vi "Actor Core.vi"(8 "error in":errorcluster, 11 "CS++MCSGui.lvclass":refnum<class "CS++MCSGui.lvclass">) -> (0 "Error Out":errorcluster, 3 "Actor out":refnum<class "Actor.lvclass">)   [LabVIEW 2016, in "CS++MCSGui.lvlib" / "CS++MCSGui.lvclass"]
doc: "(<B>Filename</B>: Actor Framework.lvlib:Actor.lvclass:Actor Core.vi)\n\nReceives messages to the actor, reacts to them, and initiates any error handling that may shut the actor down.\n\nDescendant classes may override this VI to append parallel tasks for the actor to complete while it handles messages. Overrides use the Call Parent Method node."
uses:
  CS++MCSGui.lvclass
  C:/User/Brand/LVP/CSPP-Dev/Packages/CSPP_Core/Actors/CS++BaseActor/CS++BaseActor.lvclass
  C:/User/Brand/LVP/CSPP-Dev/Packages/CSPP_Core/Actors/CS++GUIActor/CS++GUIActor.lvclass
  C:/Program Files (x86)/National Instruments/LabVIEW 2016/vi.lib/ActorFramework/Actor/Actor.lvclass
  <vilib>/ActorFramework/Actor/Actor.lvclass
  CSPP_Core/Actors/CS++BaseActor/CS++BaseActor.lvclass/CS++BaseActor.ctl
  CSPP_Core/Actors/CS++GUIActor/CS++GUIActor.lvclass/CS++GUIActor.ctl
  <vilib>/ActorFramework/Actor/Actor.lvclass/Actor.ctl
  <vilib>/ActorFramework/Message Enqueuer/Message Enqueuer.lvclass/Message Enqueuer.ctl
  CSPP_Core/Classes/CS++ProcessVariables/ProcessVariable/PV.lvclass/PV.ctl
  CSPP_Core/Actors/CS++BaseActor/Read Object Name.vi
  CSPP_Core/Actors/CS++BaseActor/Read CS++Factory.vi
  CSPP_Core/Actors/CS++GUIActor/Read Associated Actor Name.vi
  CSPP_Core/Classes/CS++ProcessVariables/ProcessVariable/Read Data.vi
  CSPP_Core/Classes/CS++ProcessVariables/ProcessVariable/Read Name.vi
  CSPP_Core/Classes/CS++ProcessVariables/ProcessVariable/Read Timestamp.vi
  CSPP_Core/Actors/CS++GUIActor/Read Stop-Event.vi
  CSPP_Core/Actors/CS++GUIActor/Read PV-Update.vi
  CSPP_Core/Actors/CS++GUIActor/Read Associated Proxy Actor Enqueuer.vi
  <vilib>/ActorFramework/Message Enqueuer/Init from Existing Queue.vi
  <vilib>/ActorFramework/Message Enqueuer/Enqueue.vi
  <vilib>/ActorFramework/Stop Msg/Stop Msg.lvclass
  C:/Program Files (x86)/National Instruments/LabVIEW 2016/vi.lib/ActorFramework/Message/Message.lvclass
  <vilib>/ActorFramework/Message Priority Queue/Priority Enqueue.vi
  CSPP_Core/Classes/CS++ProcessVariables/PVConnection/PVConnection.lvclass
  CSPP_Core/Classes/CS++BaseClasses/Factory/CS++Factory.lvclass
  CSPP_Core/Classes/CS++ProcessVariables/ProcessVariable/PV.lvclass
  <vilib>/ActorFramework/Message Enqueuer/Message Enqueuer.lvclass
  CSPP_Core/Actors/CS++DeviceGUIActor/CS++DeviceGUIActor.lvclass
  CSPP_Core/Actors/CS++BaseActor/CS++BaseActor.lvclass
  CSPP_Core/Actors/CS++GUIActor/CS++GUIActor.lvclass
  CSPP_Core/Libraries/Utilities/CS++Utilities.lvlib
panel:
  in  "Tab Control":enum32{"Info", "Configuration", "Measurement"}(tab)
  out "Last Update":timestamp
  out "Associated Device Actor":string
  out "Resource Name":string
  out "Self-Test Result Message":string
  out "Self-Test Result Code":i32
  out "Firmware Revision":string
  out "Driver Revision":string
  in  "Read Button":bool
  in  "TriggerSlope":u16(ring) items=["rising", "falling"]
  in  "DiscriminatorSlope":u16(ring) items=["rising", "falling"]
  out "Actual Bin Width":dbl[unit]
  in  "NumberOfRecords":dbl
  in  "NumberOfBins":dbl
  in  "Bin Width":dbl[unit]
  in  "Trigger Level":dbl[unit]
  in  "Discriminator Level":dbl[unit]
  in  "Read Button":bool
  out "Status":dbl
  in  "Clear Button":bool
  in  "Stop Button":bool
  in  "Start Button":bool
  out "TotalCounts":dbl
  out "Counts":dbl
  out "NumberOfBins":dbl
  out "NumberOfRecords":dbl
  out "Bin Width":dbl[unit]
  out "Waveform Graph":dbl[](graph)
  in  "Stop Button":bool
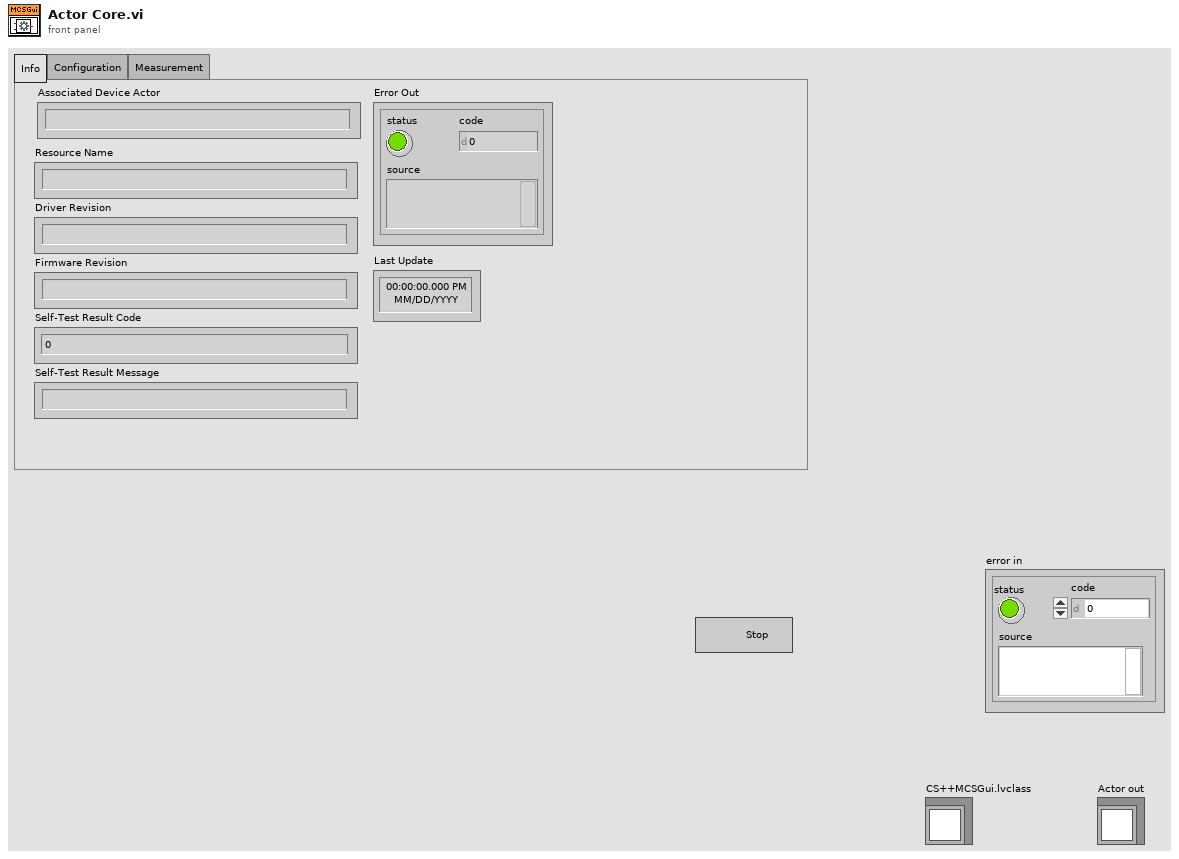
[diagram p1: front panel]
types:
  T1 = enum32{"Invalid", "Standard", "Closed", "Hidden", "Minimized", "Maximized"}
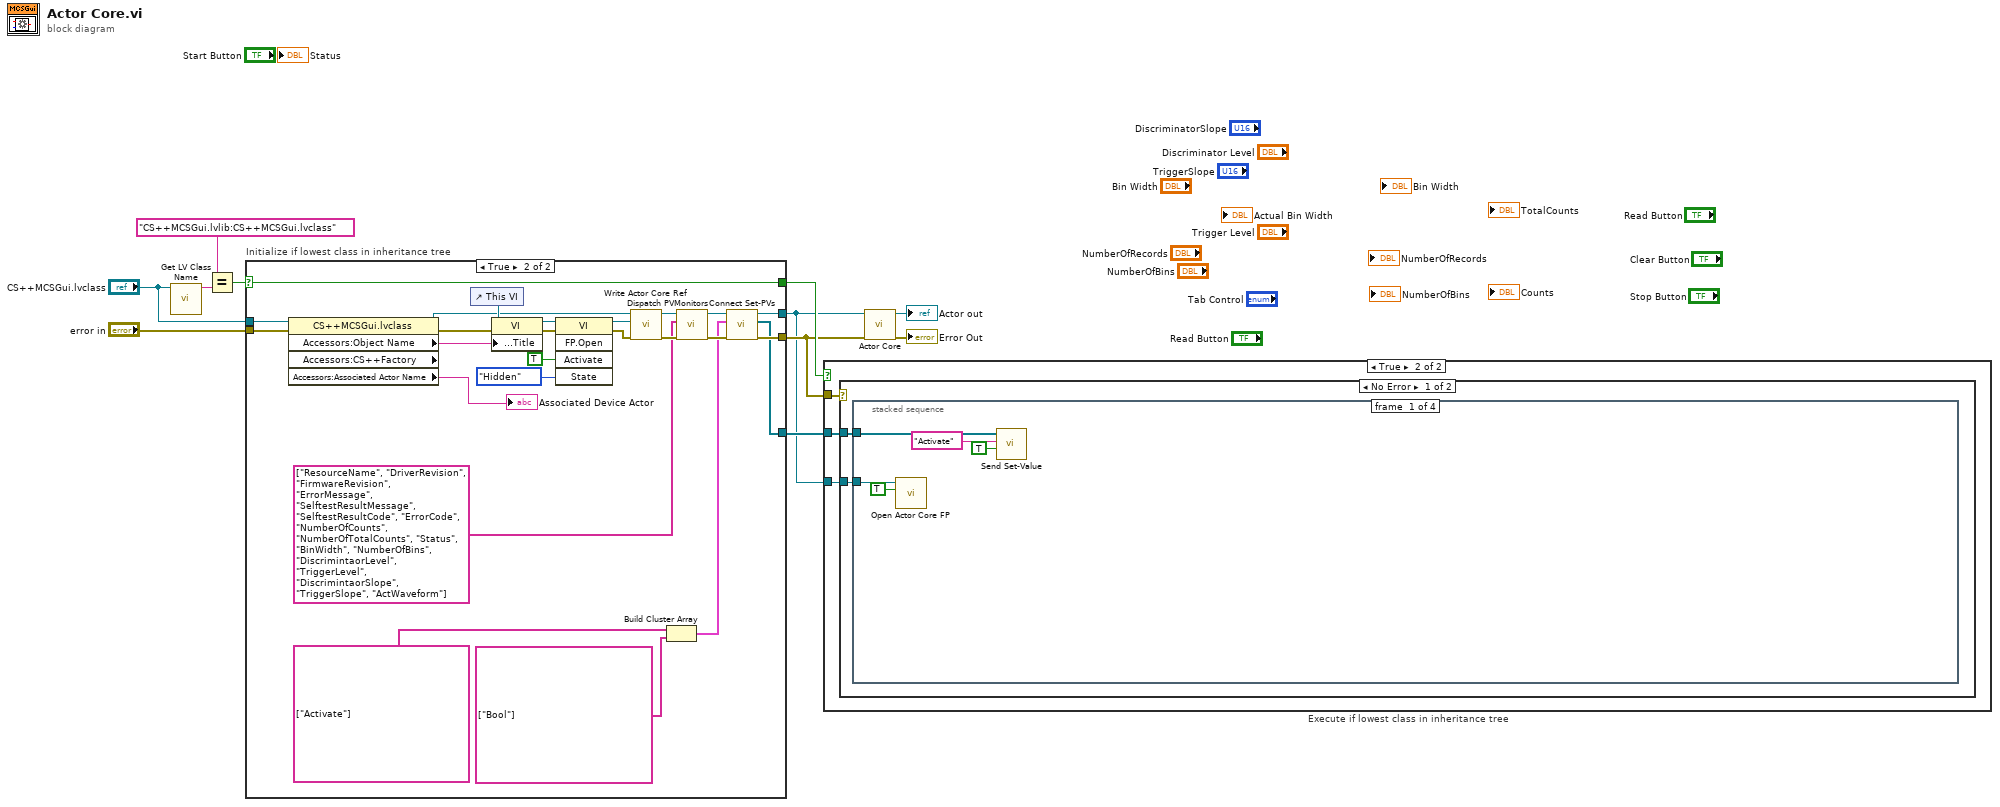
[diagram p0: block diagram]
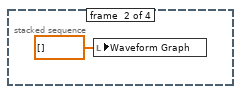
[diagram p3: hidden frame]
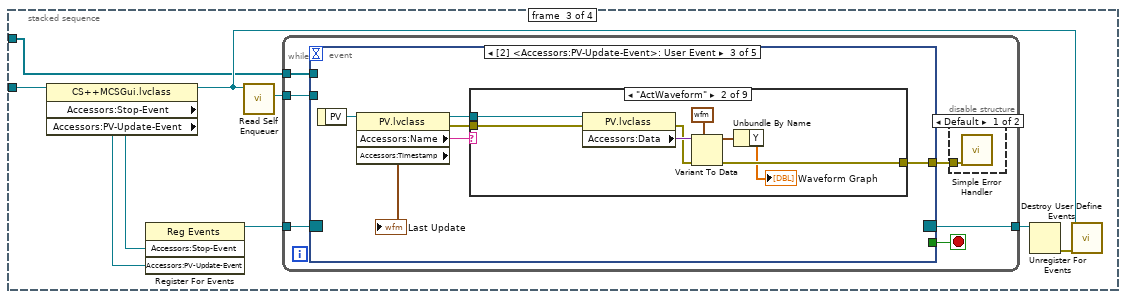
[diagram p4: hidden frame]
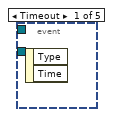
[diagram p6: hidden frame]
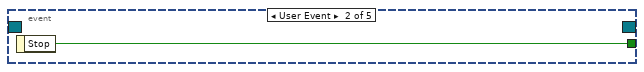
[diagram p7: hidden frame]
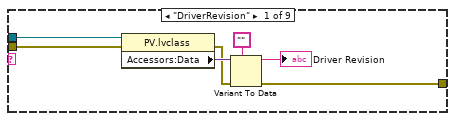
[diagram p8: hidden frame]
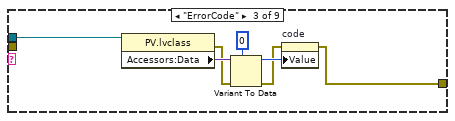
[diagram p9: hidden frame]
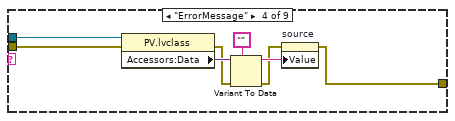
[diagram p10: hidden frame]
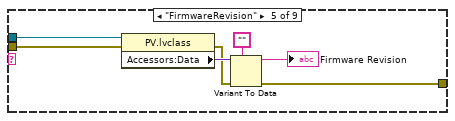
[diagram p11: hidden frame]
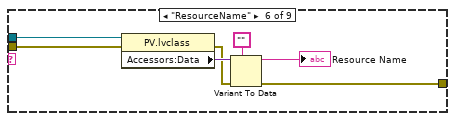
[diagram p12: hidden frame]
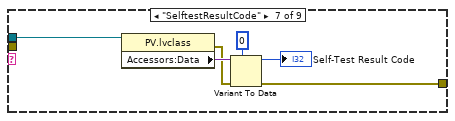
[diagram p13: hidden frame]
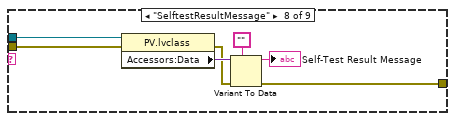
[diagram p14: hidden frame]
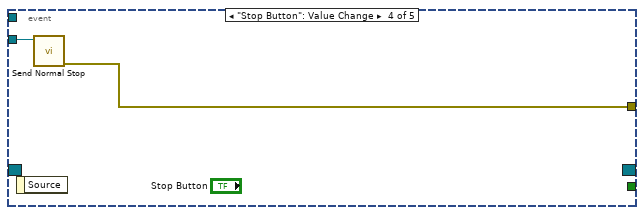
[diagram p16: hidden frame]
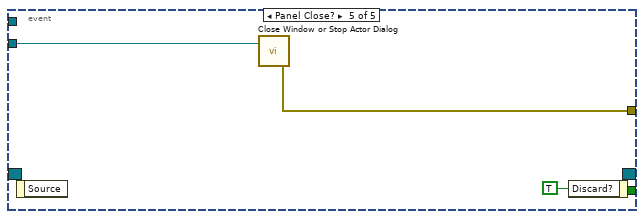
[diagram p17: hidden frame]
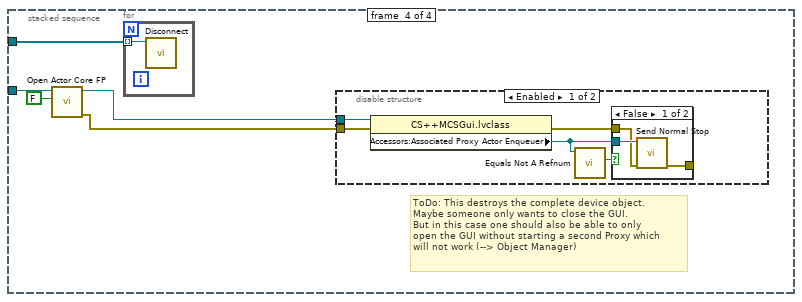
[diagram p18: hidden frame]
diagram:
  n1 = call <vilib>:"Get LV Class Name.vi"("object"="CS++MCSGui.lvclass") -> ("class name"=w10:string)  [unwired: 9 in, 1 out]
  n2 = Equal?(x="CS++MCSGui.lvlib:CS++MCSGui.lvclass" ("class name"), y=w10) -> (x = y?=w9:bool)
  n3 = case "Initialize if lowest class in inheritance tree" shown="True" w9 {
    selector: w9 -> [w14 w37]
    tunnel: "error in" -> [w12 w28]
    tunnel: "CS++MCSGui.lvclass" -> [w13 w35]
    tunnel: [w13 w23] -> w2
    tunnel: [w12 w21] -> w3
    tunnel: [w14 w37] -> w8
    tunnel: [_ w19] -> w6
    frame False {
    }
    frame True {
      n4 = property class="CS++MCSGui.lvclass" props=["Accessors:Object Name", "Accessors:CS++Factory", "Accessors:Associated Actor Name"](reference=w35, error in=w28) -> (reference out=w29:refnum<class "CS++MCSGui.lvclass">, error out=w30:errorcluster, "Accessors:Object Name"=w27:string, "Accessors:Associated Actor Name"=→"Associated Device Actor":string)  [unwired: 1 out]
      n5 = control-ref of="This VI"() -> (w33:refnum<vi>)
      n6 = property class="VI"(reference=w33, error in=w30, "Front Panel.Title"=w27) -> (reference out=w32:refnum<vi>, error out=w31:errorcluster)
      n7 = invoke class="VI" method="FP.Open"(reference=w32, error in=w31, "Activate"=TRUE ("Activate?"), "State"=T1."Hidden") -> (reference out=w36:refnum<vi>, error out=w34:errorcluster)  [unwired: 1 in, 3 out]
      n8 = call "Write Actor Core Ref.vi"("error in (no error)"=w34, "Actor Core Ref"=w36, "CS++BaseActor in"=w29) -> ("error out"=w25:errorcluster, "CS++BaseActor out"=w26:refnum<class "CS++MCSGui.lvclass">)  [unwired: 7 in]
      n9 = Build Cluster Array(string[] ["Activate"], string[] ["Bool"]) -> (w18:cluster{string, string}[])
      n10 = call "Dispatch PVMonitors.vi"("Error In"=w25, "PV Names (empty)"=string[] ["ResourceName", "DriverRevision", "FirmwareRevision", "ErrorMessage", "SelftestResultMessage", "SelftestResultCode", "ErrorCode", "NumberOfCounts", "NumberOfTotalCounts", "Status", "BinWidth", "NumberOfBins", "DiscrimintaorLevel", "TriggerLevel", "DiscrimintaorSlope", "TriggerSlope", "ActWaveform"], "CS++GUIActor in"=w26) -> ("Error Out"=w22:errorcluster, "CS++GUIActor out"=w24:refnum<class "CS++MCSGui.lvclass">)  [unwired: 7 in]
      n11 = call "Connect Set-PVs.vi"("Error In"=w22, "Set-Messages"=w18, "CS++GUIActor in"=w24) -> ("Error Out"=w21:errorcluster, "PVConnections"=w19:refnum<class "PVConnection.lvclass">[], "CS++GUIActor out"=w23:refnum<class "CS++MCSGui.lvclass">)  [unwired: 6 in]
    }
  }
  n12 = case "Execute if lowest class in inheritance tree" shown="True" w8 {
    tunnel: w2 -> [_ w42]
    tunnel: w3 -> [_ w41]
    tunnel: w6 -> [_ w40]
    frame False {
    }
    frame True {
      n13 = case shown="No Error" w41 {
        tunnel: w42 -> [w44 _]
        tunnel: w40 -> [w43 _]
        frame No Error {
          n14 = stacked-sequence {
            tunnel: w44 -> [w49 _ w56 w141]
            tunnel: w43 -> [w47 _ w51 w139]
            frame #0 {
              n15 = call "Open Actor Core FP.vi"("Open FP (F)"=TRUE, "CS++BaseActor in"=w49) -> ()  [unwired: 8 in, 2 out]
              n16 = call "Send Set-Value.vi"("Data"=TRUE ("Open FP (F)"), "PVName"="Activate", "PVConnections"=w47) -> ()  [unwired: 7 in, 2 out]
            }
            frame #1 {
              n17 = local write "Waveform Graph"(dbl[] [] ("Waveform Graph")) -> ()
            }
            frame #2 {
              n18 = property class="CS++MCSGui.lvclass"(reference=w56) -> (reference out=w55:refnum<class "CS++MCSGui.lvclass">, "Accessors:Stop-Event"=w53:refnum<user-event>, "Accessors:PV-Update-Event"=w52:refnum<user-event>)  [unwired: 1 in, 1 out]
              n19 = register-events(w53, w52) -> (reference out=w54:refnum<event-registration>)  [unwired: 2 in, 1 out]
              n20 = call <vilib>:"Read Self Enqueuer.vi"("Actor"=w55) -> ("Self Enqueuer"=w57:refnum<class "Message Enqueuer.lvclass">)  [unwired: 10 in]
              n21 = while {
                tunnel: w54 -> [w65]
                tunnel: [w63] -> w59
                tunnel: w57 -> [w61]
                tunnel: w51 -> [w60]
                stop <- w64 stop-if-true
                n22 = event shown="[2] <Accessors:PV-Update-Event>: User Event" {
                  selector: w65 -> [_ _ _ _ _]
                  dyn-events: [_ _ _ _ _] -> w63
                  timeout: _ -> [_ _ _ _ _]
                  tunnel: [_ w67 _ _ _] -> w64
                  tunnel: [_ _ w69 w133 w134] -> w62
                  tunnel: w61 -> [_ _ _ w132 w135]
                  tunnel: w60 -> [_ _ _ _ _]
                  event Timeout {
                    n23 = event-data() -> ()  [unwired: 1 in, 2 out]
                  }
                  event User Event {
                    n24 = event-data() -> ("Stop"=w67:bool)  [unwired: 1 in]
                  }
                  event User Event {
                    n25 = event-data() -> ("PV"=w70:refnum<class "PV.lvclass">)  [unwired: 1 in]
                    n26 = property class="PV.lvclass"(reference=w70) -> (reference out=w71:refnum<class "PV.lvclass">, error out=w72:errorcluster, "Accessors:Name"=w73:string, "Accessors:Timestamp"=→"Last Update":timestamp)  [unwired: 1 in]
                    n27 = case shown="\"ActWaveform\"" w73 {
                      tunnel: w71 -> [w78 w87 w93 w101 w108 w115 w121 w128 _]
                      tunnel: w72 -> [w77 w86 _ w100 w107 w114 _ w127 w131]
                      tunnel: [w75 w84 w90 w96 w105 w112 w120 w125 w131] -> w69
                      frame "DriverRevision" {
                        n28 = property class="PV.lvclass"(reference=w78, error in=w77) -> (error out=w76:errorcluster, "Accessors:Data"=w79:variant)  [unwired: 1 out]
                        n29 = Variant To Data(error in=w76, type="", Variant=w79) -> (data=→"Driver Revision":string, error out=w75:errorcluster)
                      }
                      frame "ActWaveform" {
                        n30 = property class="PV.lvclass"(reference=w87, error in=w86) -> (error out=w85:errorcluster, "Accessors:Data"=w88:variant)  [unwired: 1 out]
                        n31 = Variant To Data(error in=w85, type=waveform(dbl) {"t0"=timestamp(0 s since 1904-01-01), "dt"=1.0, "Y"=[]} ("Waveform Data"), Variant=w88) -> (data=w82:waveform(dbl), error out=w84:errorcluster)
                        n32 = Unbundle By Name(w82) -> ("Y"=→"Waveform Graph":dbl[])
                      }
                      frame "ErrorCode" {
                        n33 = property class="PV.lvclass"(reference=w93) -> (error out=w89:errorcluster, "Accessors:Data"=w94:variant)  [unwired: 1 in, 1 out]
                        n34 = Variant To Data(error in=w89, type=0, Variant=w94) -> (data=w92:i32, error out=w91:errorcluster)
                        n35 = property on="code" class="DigNum (strict)"(error in=w91, "Value"=w92) -> (error out=w90:errorcluster)  [unwired: 1 in, 1 out]
                      }
                      frame "ErrorMessage" {
                        n36 = property class="PV.lvclass"(reference=w101, error in=w100) -> (error out=w99:errorcluster, "Accessors:Data"=w102:variant)  [unwired: 1 out]
                        n37 = Variant To Data(error in=w99, type="", Variant=w102) -> (data=w98:string, error out=w97:errorcluster)
                        n38 = property on="source" class="Str"(error in=w97, "Value"=w98) -> (error out=w96:errorcluster)  [unwired: 1 in, 1 out]
                      }
                      frame "FirmwareRevision" {
                        n39 = property class="PV.lvclass"(reference=w108, error in=w107) -> (error out=w106:errorcluster, "Accessors:Data"=w109:variant)  [unwired: 1 out]
                        n40 = Variant To Data(error in=w106, type="", Variant=w109) -> (data=→"Firmware Revision":string, error out=w105:errorcluster)
                      }
                      frame "ResourceName" {
                        n41 = property class="PV.lvclass"(reference=w115, error in=w114) -> (error out=w113:errorcluster, "Accessors:Data"=w116:variant)  [unwired: 1 out]
                        n42 = Variant To Data(error in=w113, type="", Variant=w116) -> (data=→"Resource Name":string, error out=w112:errorcluster)
                      }
                      frame "SelftestResultCode" {
                        n43 = property class="PV.lvclass"(reference=w121) -> (error out=w119:errorcluster, "Accessors:Data"=w122:variant)  [unwired: 1 in, 1 out]
                        n44 = Variant To Data(error in=w119, type=0, Variant=w122) -> (data=→"Self-Test Result Code":i32, error out=w120:errorcluster)
                      }
                      frame "SelftestResultMessage" {
                        n45 = property class="PV.lvclass"(reference=w128, error in=w127) -> (error out=w126:errorcluster, "Accessors:Data"=w129:variant)  [unwired: 1 out]
                        n46 = Variant To Data(error in=w126, type="", Variant=w129) -> (data=→"Self-Test Result Message":string, error out=w125:errorcluster)
                      }
                      frame Default {
                      }
                    }
                  }
                  event "Stop Button": Value Change {
                    n47 = event-data() -> ()  [unwired: 1 in, 1 out]
                    n48 = call <vilib>:"Send Normal Stop.vi"("Message Enqueuer"=w132) -> ("error out"=w133:errorcluster)  [unwired: 10 in]
                  }
                  event Panel Close? {
                    n49 = event-data() -> ()  [unwired: 1 in, 1 out]
                    n50 = call "Close Window or Stop Actor Dialog.vi"("Self Enqueuer"=w135) -> ("Error Out"=w134:errorcluster)  [unwired: 2 in]
                    n51 = event-data("Discard?"=TRUE) -> ()  [unwired: 1 in, 1 out]
                  }
                }
                n52 = disable-structure shown="Default" {
                  disable-tunnel: w62 -> [w66 _]
                  frame condition #0 (active) {
                    n53 = call <vilib>:"Simple Error Handler.vi"("error in (no error)"=w66) -> ()  [unwired: 4 in, 5 out]
                  }
                  frame condition #1 {
                  }
                }
              }
              n54 = Unregister For Events(event registration refnum=w59) -> (error out=w58:errorcluster)  [unwired: 1 in]
              n55 = call-dynamic "Destroy User Define Events.vi"("error in (no error)"=w58, "CS++GUIActor in"=w55) -> ()  [unwired: 8 in, 2 out]
            }
            frame #3 {
              # "ToDo: This destroys the complete device object.\nMaybe someone only wants to close the GUI. \nBut in this case one should also be able to only \nopen the GUI without starting a second Proxy which\nwill not work (--> Object Manager)"
              n56 = call "Open Actor Core FP.vi"("Open FP (F)"=FALSE, "CS++BaseActor in"=w141) -> ("error out"=w137:errorcluster, "CS++BaseActor out"=w138:refnum<class "CS++MCSGui.lvclass">)  [unwired: 8 in]
              n57 = for {
                tunnel: w139 -> [w151] mode=indexing
                n58 = call "Disconnect.vi"("PVConnection in"=w151) -> ()  [unwired: 9 in, 2 out]
              }
              n59 = disable-structure shown="Enabled" {
                disable-tunnel: w138 -> [w146 _]
                disable-tunnel: w137 -> [w142 _]
                frame Enabled {
                  n60 = property class="CS++MCSGui.lvclass"(reference=w146, error in=w142) -> (error out=w145:errorcluster, "Accessors:Associated Proxy Actor Enqueuer"=w144:refnum<class "Message Enqueuer.lvclass">)  [unwired: 1 out]
                  n61 = call <vilib>:"Equals Not A Refnum.vi"("Message Enqueuer"=w144) -> ("Not a refnum?"=w143:bool)  [unwired: 10 in]
                  n62 = case shown="False" w143 {
                    tunnel: [w149 w150] -> _
                    tunnel: w144 -> [w148 _]
                    tunnel: w145 -> [w147 w150]
                    frame False {
                      n63 = call <vilib>:"Send Normal Stop.vi"("error in (no error)"=w147, "Message Enqueuer"=w148) -> ("error out"=w149:errorcluster)  [unwired: 9 in]
                    }
                    frame True {
                    }
                  }
                }
                frame Disabled {
                }
              }
            }
          }
        }
        frame Error {
        }
      }
    }
  }
  n64 = call-parent "Actor Core.vi"("error in"=w3, "CS++DeviceGUIActor.lvclass"=w2) -> ("Error Out"=→"Error Out":errorcluster, "Actor out"=→"Actor out":refnum<class "Actor.lvclass">)  [unwired: 8 in]
